vi "thres_conf_ASIC.vi"(6 "threshold":u32, 7 "Ring":u16(ring)=5 items=["Channel 0", "Channel 1", "Channel 2", "Channel 3", "Channel 4", "Channel 5", "Channel 6"], 8 "error out 3":errorcluster, 10 "Id in":i32, 11 "connection ID":refnum<k5>) -> (0 "error out 2":errorcluster, 2 "data read value":u32, 3 "connection ID out":refnum<k5>, 5 "Id out":i32=72)   [LabVIEW 2012]
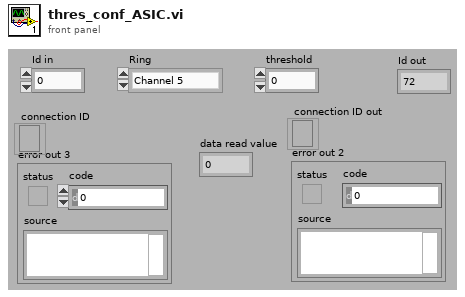
[diagram p1: front panel]
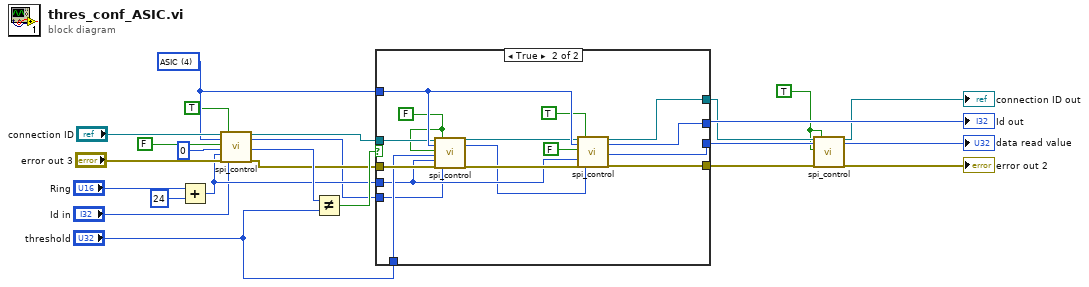
[diagram p0: block diagram]
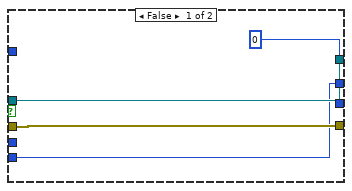
[diagram p2: hidden frame]
diagram:
  w1 = TRUE ("Read/#write")
  w19 = u16 4 items=["Attenuation", "Clipping", "Enable channel", "Delay line", "ASIC"] ("Device")
  n1 = Add(x="Ring", y=u16 24) -> (x+y=w10:u16)
  n2 = call "spi_control.vi"("connection ID"="connection ID", "Device"=w19, "Read/#write"=FALSE, "Data"=0, "Register or channel"=w10, "error in"="error out 3", "Read physical"=TRUE, "Id in"="Id in") -> ("connection ID out"=w18:refnum<k5>, "Id out"=w9:i32, "data read value"=w21:u32, "error out 2"=w17:errorcluster)  [unwired: 4 in, 4 out]
  n3 = Not Equal?(x=w21, y="threshold") -> (x != y?=w20:bool)
  n4 = case shown="True" w20 {
    tunnel: w19 -> [_ w43]
    tunnel: w18 -> [w27 w41]
    tunnel: w17 -> [w26 w40]
    tunnel: "threshold" -> [_ w38]
    tunnel: w10 -> [_ w37]
    tunnel: w9 -> [w25 w32]
    tunnel: [w26 w31] -> w5
    tunnel: [w27 w30] -> w3
    tunnel: [0 ("Id out") w29] -> w8
    tunnel: [w25 w28] -> w7
    frame False {
    }
    frame True {
      w34 = FALSE ("Read physical")
      n5 = call "spi_control.vi"("connection ID"=w41, "Device"=w43, "Read/#write"=w34, "Data"=w38, "Register or channel"=w37, "error in"=w40, "Read physical"=w34, "Id in"=w32) -> ("connection ID out"=w42:refnum<k5>, "Id out"=w33:i32, "error out 2"=w39:errorcluster)  [unwired: 4 in, 5 out]
      n6 = call "spi_control.vi"("connection ID"=w42, "Device"=w43, "Read/#write"=FALSE, "Register or channel"=w37, "error in"=w39, "Read physical"=TRUE, "Id in"=w33) -> ("connection ID out"=w30:refnum<k5>, "Id out"=w28:i32, "data read value"=w29:u32, "error out 2"=w31:errorcluster)  [unwired: 5 in, 4 out]
    }
  }
  "Id out" <- w7
  "data read value" <- w8
  n7 = call "spi_control.vi"("connection ID"=w3, "Read/#write"=w1, "error in"=w5, "Read physical"=w1) -> ("connection ID out"=→"connection ID out":refnum<k5>, "error out 2"=→"error out 2":errorcluster)  [unwired: 8 in, 6 out]
